vi "Run_All_Tests.vi"() -> ()   [LabVIEW 2019]
panel:
  out "Packet":bool
  out "PhotonCamera":bool
  out "All Tests Finished":bool
  out "PhotonVisionUtil":bool
  # "FORMAL PHOTON VISION LIB LIBRARY TEST PROCEDURE"
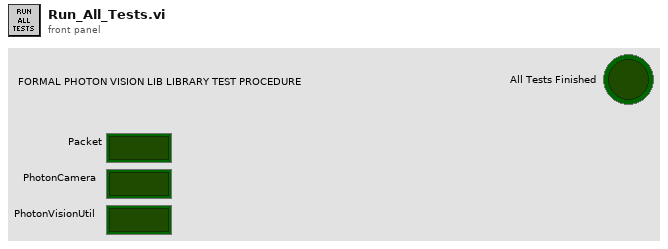
[diagram p1: front panel]
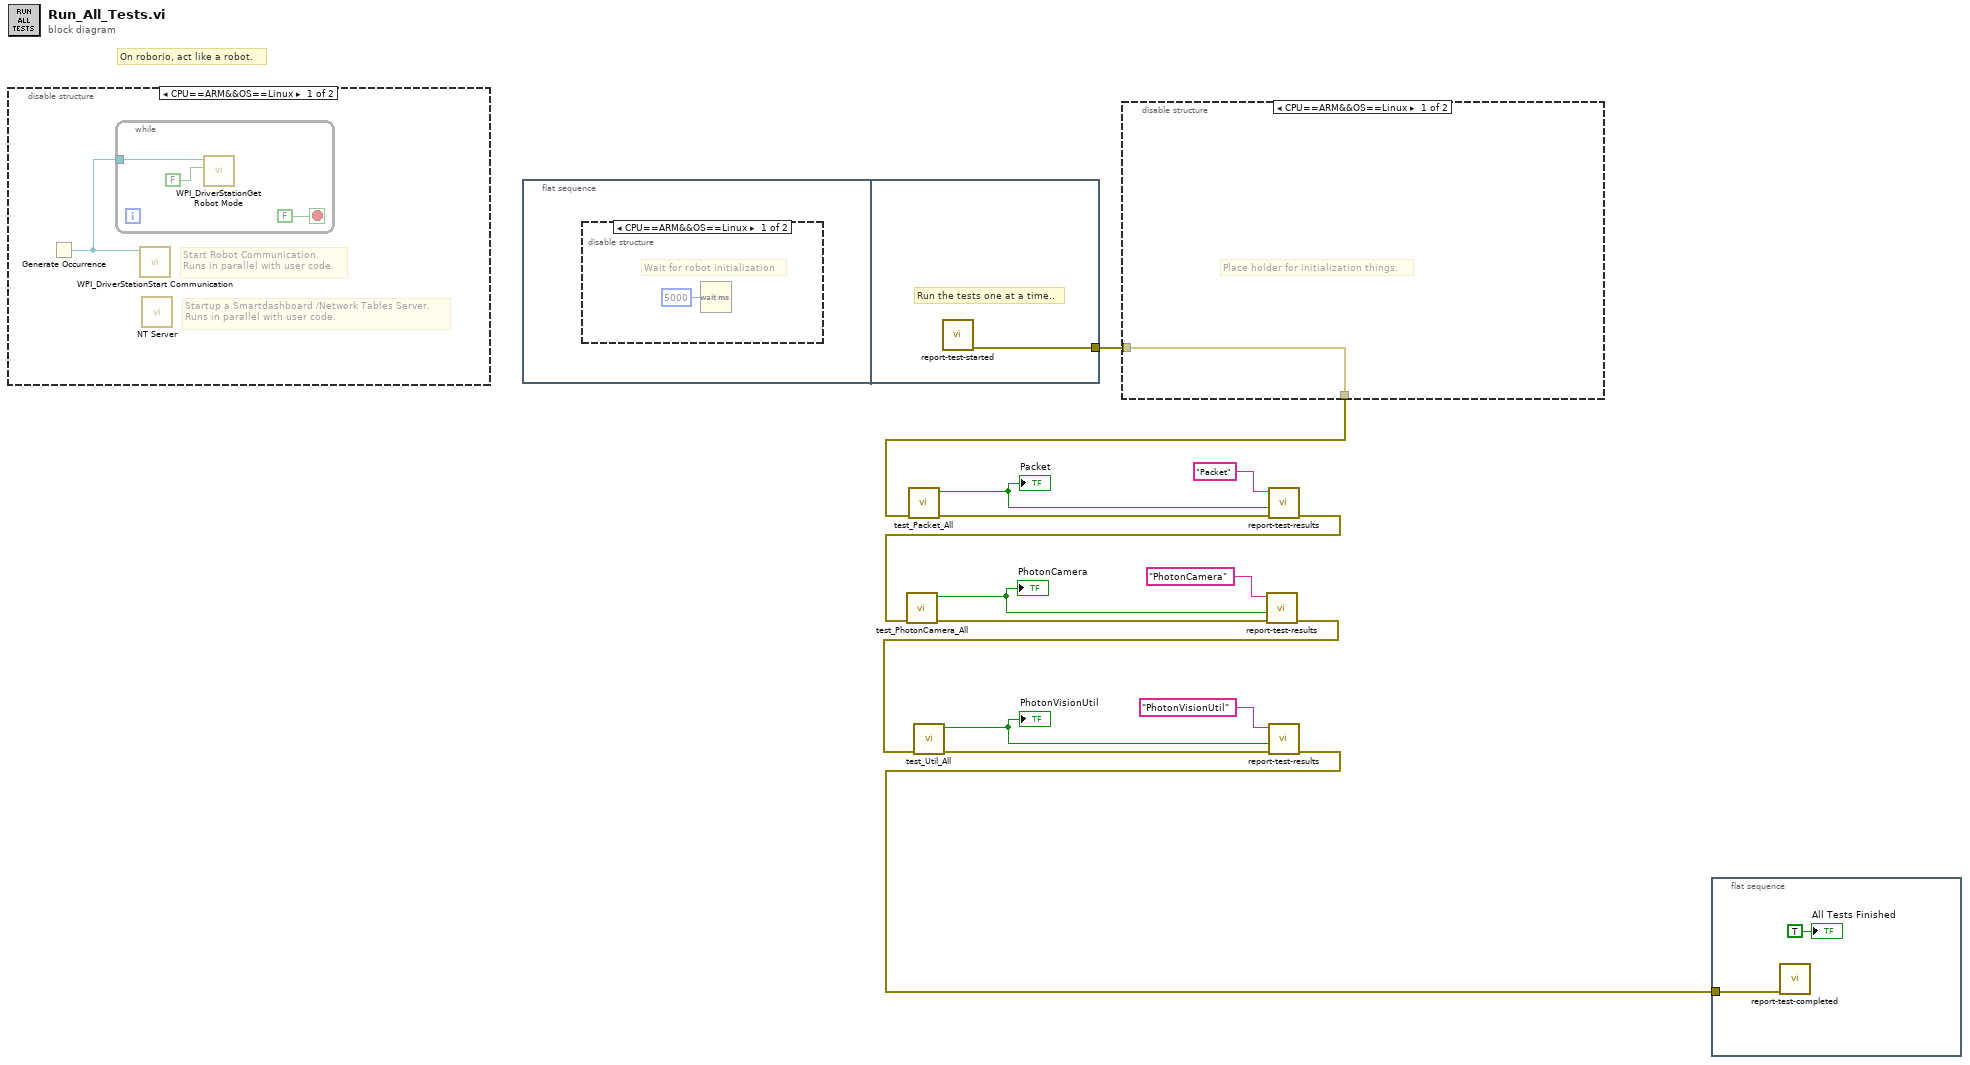
[diagram p0: block diagram]
diagram:
  # "On roborio, act like a robot."
  n1 = disable-structure shown="CPU==ARM&&OS==Linux" {
    frame condition #0 {
      # "Startup a Smartdashboard /Network Tables Server.\nRuns in parallel with user code."
      # "Start Robot Communication.\nRuns in parallel with user code."
      n2 = Generate Occurrence() -> (w15:refnum<k4>)
      n3 = while {
        tunnel: w15 -> [w18]
        stop <- FALSE stop-if-true
        n4 = call <vilib>:"WPI_DriverStationGet Robot Mode.vi"("Finish"=FALSE, "DS Occurrence"=w18) -> ()  [unwired: 10 out]
      }
      n5 = call <vilib>:"WPI_DriverStationStart Communication.vi"("occurrence"=w15) -> ()  [unwired: 2 in, 9 out]
      n6 = call <vilib>:"NT Server.vi"() -> ()  [unwired: 12 in]
    }
    frame condition #1 (active) {
    }
  }
  n7 = flat-sequence {
    tunnel: [w20] -> w13
    frame #0 {
      n8 = disable-structure shown="CPU==ARM&&OS==Linux" {
        frame condition #0 {
          # "Wait for robot initialization"
          n9 = Wait (ms)(milliseconds to wait=u32 5000) -> ()  [unwired: 1 out]
        }
        frame condition #1 (active) {
        }
      }
    }
    frame #1 {
      # "Run the tests one at a time.."
      n10 = call "report-test-started.vi"() -> ("error out"=w20:errorcluster)  [unwired: 11 in]
    }
  }
  n11 = disable-structure shown="CPU==ARM&&OS==Linux" {
    disable-tunnel: w13 -> [w21 w22]
    disable-tunnel: [w21 w22] -> w2
    frame condition #0 {
      # "Place holder for initialization things."
    }
    frame condition #1 (active) {
    }
  }
  n12 = call "test_Packet_All.vi"("error in (no error)"=w2) -> ("error out"=w4:errorcluster, "Test Passed"=w3:bool)  [unwired: 9 in]
  "Packet" <- w3
  n13 = call "report-test-results.vi"("error in (no error)"=w4, "TestPassed"=w3, "Test Name"="Packet") -> ("error out"=w1:errorcluster)  [unwired: 8 in]
  n14 = call "test_PhotonCamera_All.vi"("error in (no error)"=w1) -> ("error out"=w7:errorcluster, "Test Passed"=w6:bool)  [unwired: 9 in]
  "PhotonCamera" <- w6
  n15 = call "report-test-results.vi"("error in (no error)"=w7, "TestPassed"=w6, "Test Name"="PhotonCamera") -> ("error out"=w8:errorcluster)  [unwired: 8 in]
  n16 = call "test_Util_All.vi"("error in (no error)"=w8) -> ("error out"=w11:errorcluster, "Test Passed"=w10:bool)  [unwired: 9 in]
  "PhotonVisionUtil" <- w10
  n17 = call "report-test-results.vi"("error in (no error)"=w11, "TestPassed"=w10, "Test Name"="PhotonVisionUtil") -> ("error out"=w12:errorcluster)  [unwired: 8 in]
  n18 = flat-sequence {
    tunnel: w12 -> [w23]
    frame #0 {
      n19 = call "report-test-completed.vi"("error in (no error)"=w23) -> ()  [unwired: 10 in, 1 out]
      "All Tests Finished" <- TRUE ("All Tests Finished")
    }
  }
